vi "Shoot Manual and Auto Management.vi"(0 "Pilot X":dbl, 1 "Pilot Y":dbl, 2 "Elevation":dbl, 3 "Shoot Motors":dbl, 4 "Auto Shoot?":bool, 5 "Le Fire At Will":bool) -> (16 "X Drive Arcade":dbl, 17 "Y Drive Arcade":dbl)   [LabVIEW 2012]
uses:
  Motors Values.vi
  BotStatus.vi
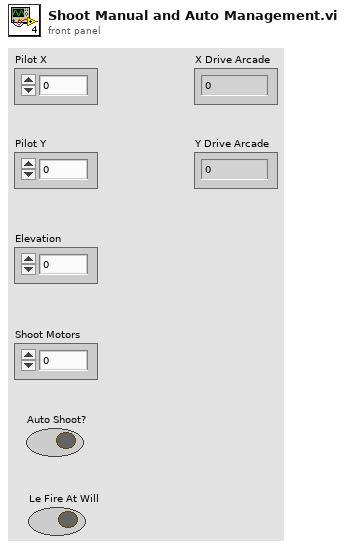
[diagram p1: front panel]
types:
  T1 = cluster{"Middle":bool, "InCannon":bool, "InFlipper":bool, "FlipperAtPlace":bool, "Bottom":bool, "FrisbeeDirection":bool}
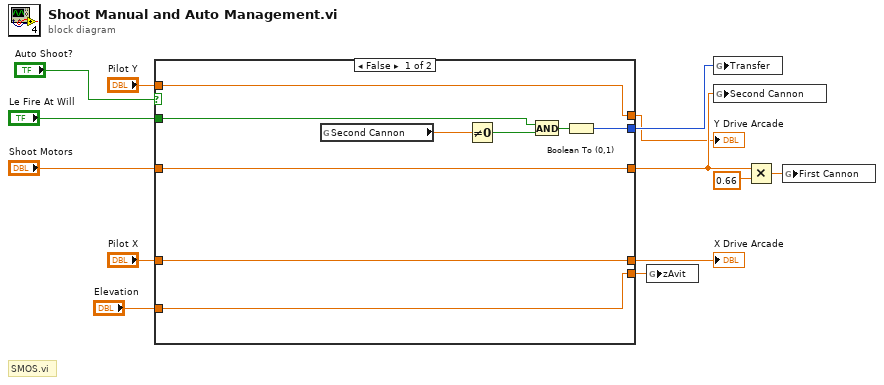
[diagram p0: block diagram]
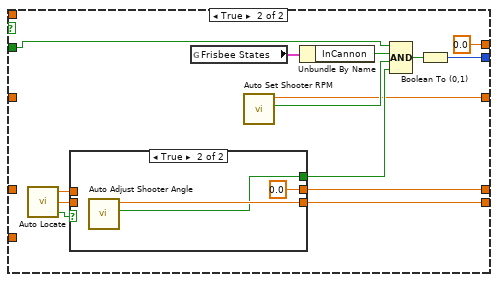
[diagram p2: hidden frame]
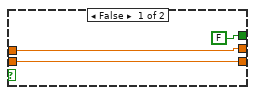
[diagram p3: hidden frame]
diagram:
  # "SMOS.vi"
  n1 = case shown="False" "Auto Shoot?" {
    tunnel: [w21 w32] -> w10
    tunnel: [w22 w33] -> w11
    tunnel: "Pilot X" -> [w22 _]
    tunnel: "Elevation" -> [w21 _]
    tunnel: "Le Fire At Will" -> [w18 w27]
    tunnel: [w16 w25] -> w7
    tunnel: [w15 w24] -> w4
    tunnel: "Shoot Motors" -> [w15 _]
    tunnel: "Pilot Y" -> [w14 _]
    tunnel: [w14 0.0] -> w1
    frame False {
      n2 = global read "Motors Values.vi" "Second Cannon"() -> (w20:dbl)
      n3 = Not Equal To 0?(x=w20) -> (x != 0?=w19:bool)
      n4 = And(x=w18, y=w19) -> (x .and. y?=w17:bool)
      n5 = Boolean To (0,1)(Boolean=w17) -> (0, 1=w16:i16)
    }
    frame True {
      n6 = call "Auto Locate.vi"() -> ("Located"=w36:bool, "zAvit"=w34:dbl, "X Drive Arcade"=w35:dbl)  [unwired: 3 in]
      n7 = case shown="True" w36 {
        tunnel: w35 -> [w38 _]
        tunnel: w34 -> [w39 _]
        tunnel: [w39 w41] -> w32
        tunnel: [w38 0.0] -> w33
        tunnel: [FALSE w40] -> w31
        frame False {
        }
        frame True {
          n8 = call "Auto Adjust Shooter Angle.vi"() -> ("On Target"=w40:bool, "zAvit Vbus Out"=w41:dbl)  [unwired: 10 in]
        }
      }
      n9 = global read "BotStatus.vi" "Frisbee States"() -> (w29:T1)
      n10 = call "Auto Set Shooter RPM.vi"() -> ("READY!"=w30:bool, "Vbus Out"=w24:dbl)  [unwired: 10 in]
      n11 = Unbundle By Name(w29) -> ("InCannon"=w28:bool)
      n12 = Compound Arithmetic op=AND(w27, w28, w30, w31) -> (w26:bool)
      n13 = Boolean To (0,1)(Boolean=w26) -> (0, 1=w25:i16)
    }
  }
  "X Drive Arcade" <- w11
  "Y Drive Arcade" <- w1
  n14 = global write "Motors Values.vi" "zAvit"(w10) -> ()
  n15 = global write "Motors Values.vi" "Transfer"(w7) -> ()
  n16 = global write "Motors Values.vi" "Second Cannon"(w4) -> ()
  n17 = Multiply(x=w4, y=0.66) -> (x*y=w5:dbl)
  n18 = global write "Motors Values.vi" "First Cannon"(w5) -> ()
